vi "一体站流程质控自动启动.vi"(6 "CODMn量程切换":enum32{"H", "L", "AUTO"}(ring)=enum."AUTO", 8 "总磷量程切换":enum32{"H", "L", "AUTO"}(ring)=enum."AUTO", 9 "总氮量程切换":enum32{"H", "L", "AUTO"}(ring)=enum."AUTO", 10 "氨氮量程切换":enum32{"H", "L", "AUTO"}(ring)=enum."AUTO", 11 "参数":T1={"是否启用仪器"=FALSE, "CODMn"={"启动测量模式"={"测量模式"=enum."水样测量"}, "确定按钮"=TRUE}, "启动模块"={"氨氮"=FALSE, "总磷"=FALSE, "总氮"=FALSE, "COD"=FALSE}, "常规启动"=FALSE, "直接启动"=FALSE}) -> ()   [LabVIEW 2016, in "质控单元.lvlib"]
uses:
  PLC/PLC.lvlib
panel:
  out "枚举 2":enum16{"初始化", "采配水启动", "等待", "配水", "排水", "结束"}(ring)
  out "枚举":enum16{"初始化", "采配水启动", "等待", "配水", "排水", "结束"}(ring)
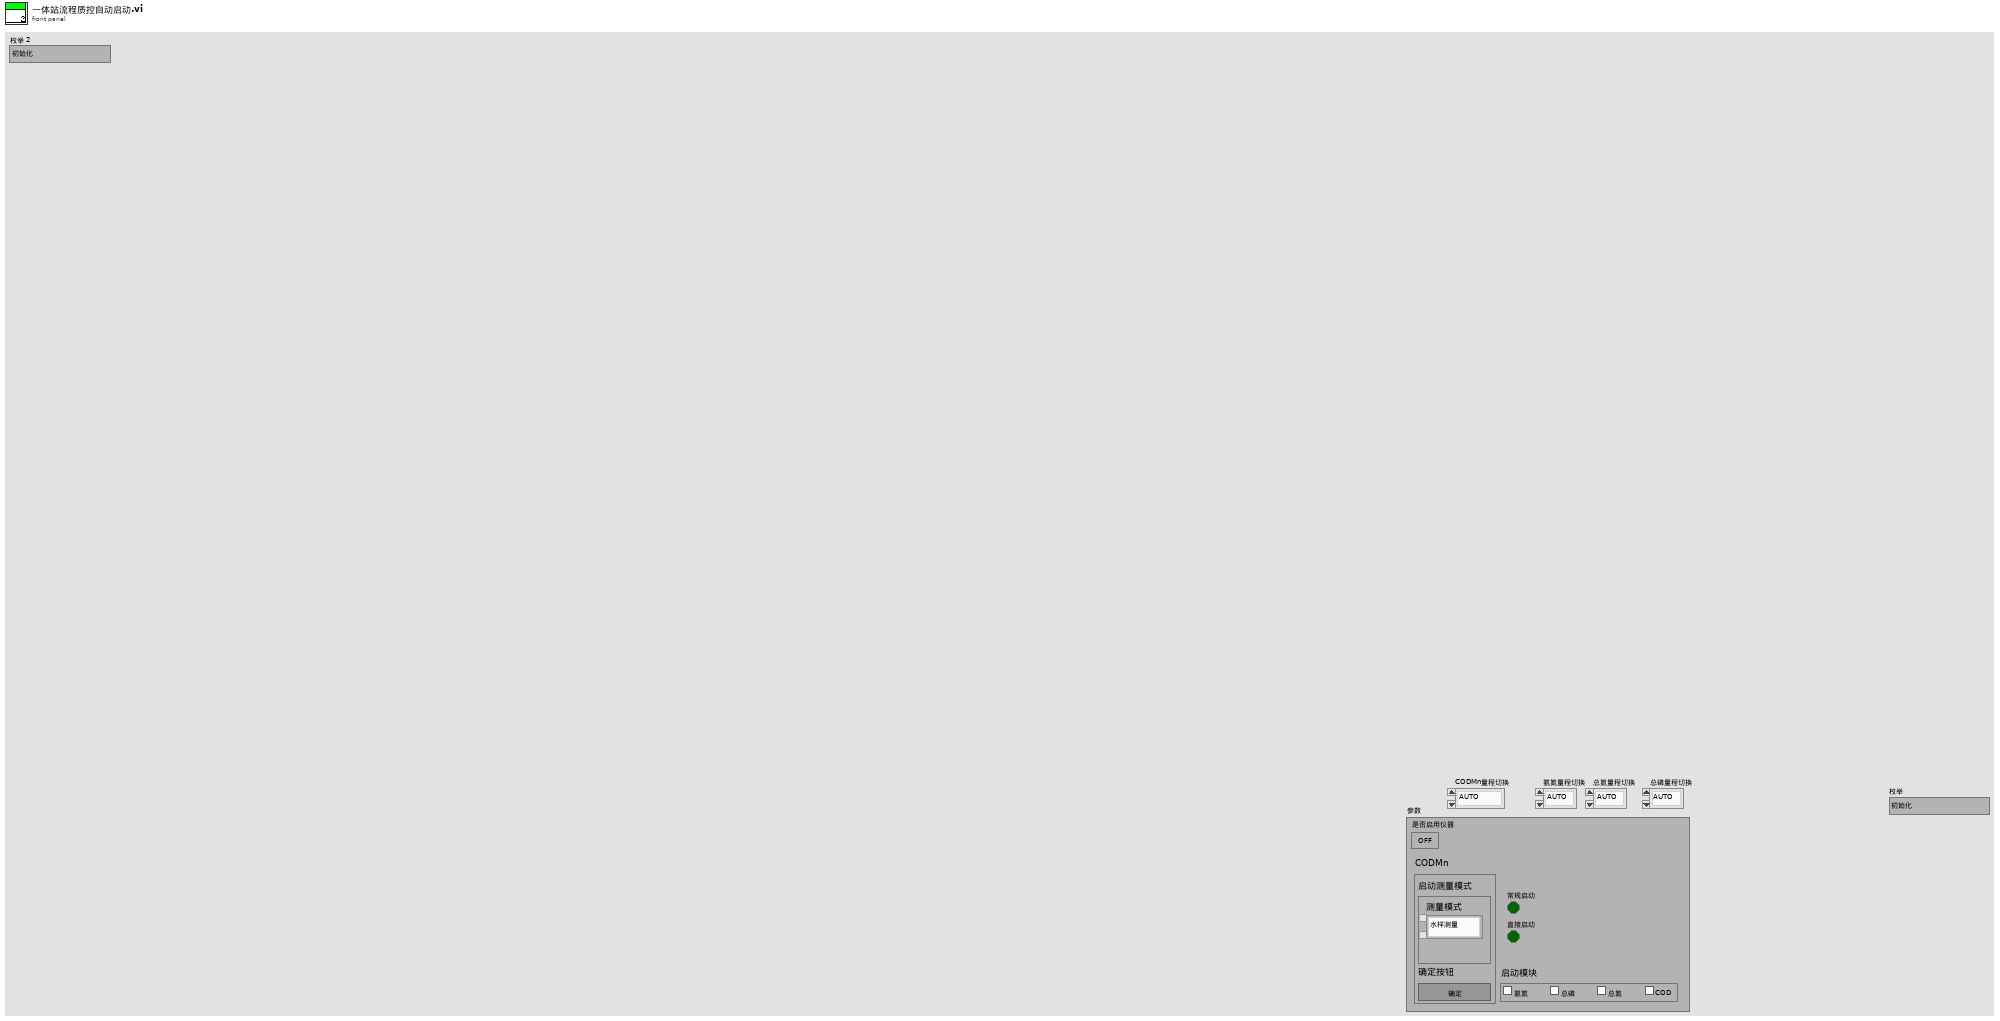
[diagram p1: front panel]
types:
  T1 = cluster{"是否启用仪器":bool, "CODMn":cluster{"启动测量模式":cluster{"测量模式":enum16{"水样测量", "标样核查", "加标回收", "平行样", "校零", "校标"}}, "确定按钮":bool}, "启动模块":cluster{"氨氮":bool, "总磷":bool, "总氮":bool, "COD":bool}, "常规启动":bool, "直接启动":bool}
  T2 = cluster{"命令":string, cluster{"starting address":u16, "holding register value":u16}}
  T3 = cluster{"R0":i16, "R1":i16, "R2":i16, "R3":i16, "R4":i16, "R5":i16, "R6":i16, "R7":i16, "R8":i16, "R9":i16, "R10":i16, "R11":i16, "R12":i16, "R13":i16, "R14":i16, "R15":i16, "R16":i16, "R17":i16, "R18":i16, "R19":i16, "R20":i16, "R21":i16, "R22":i16, "R23":i16, "R24":i16, "R25":i16, "R26":i16, "R27":i16, "R28":i16, "R29":i16, "R30":i16, "R31":i16, "R32":i16, "R33":i16, "R34":i16}
  T4 = enum32{"Bad", "Idle", "Run top level", "Running"}
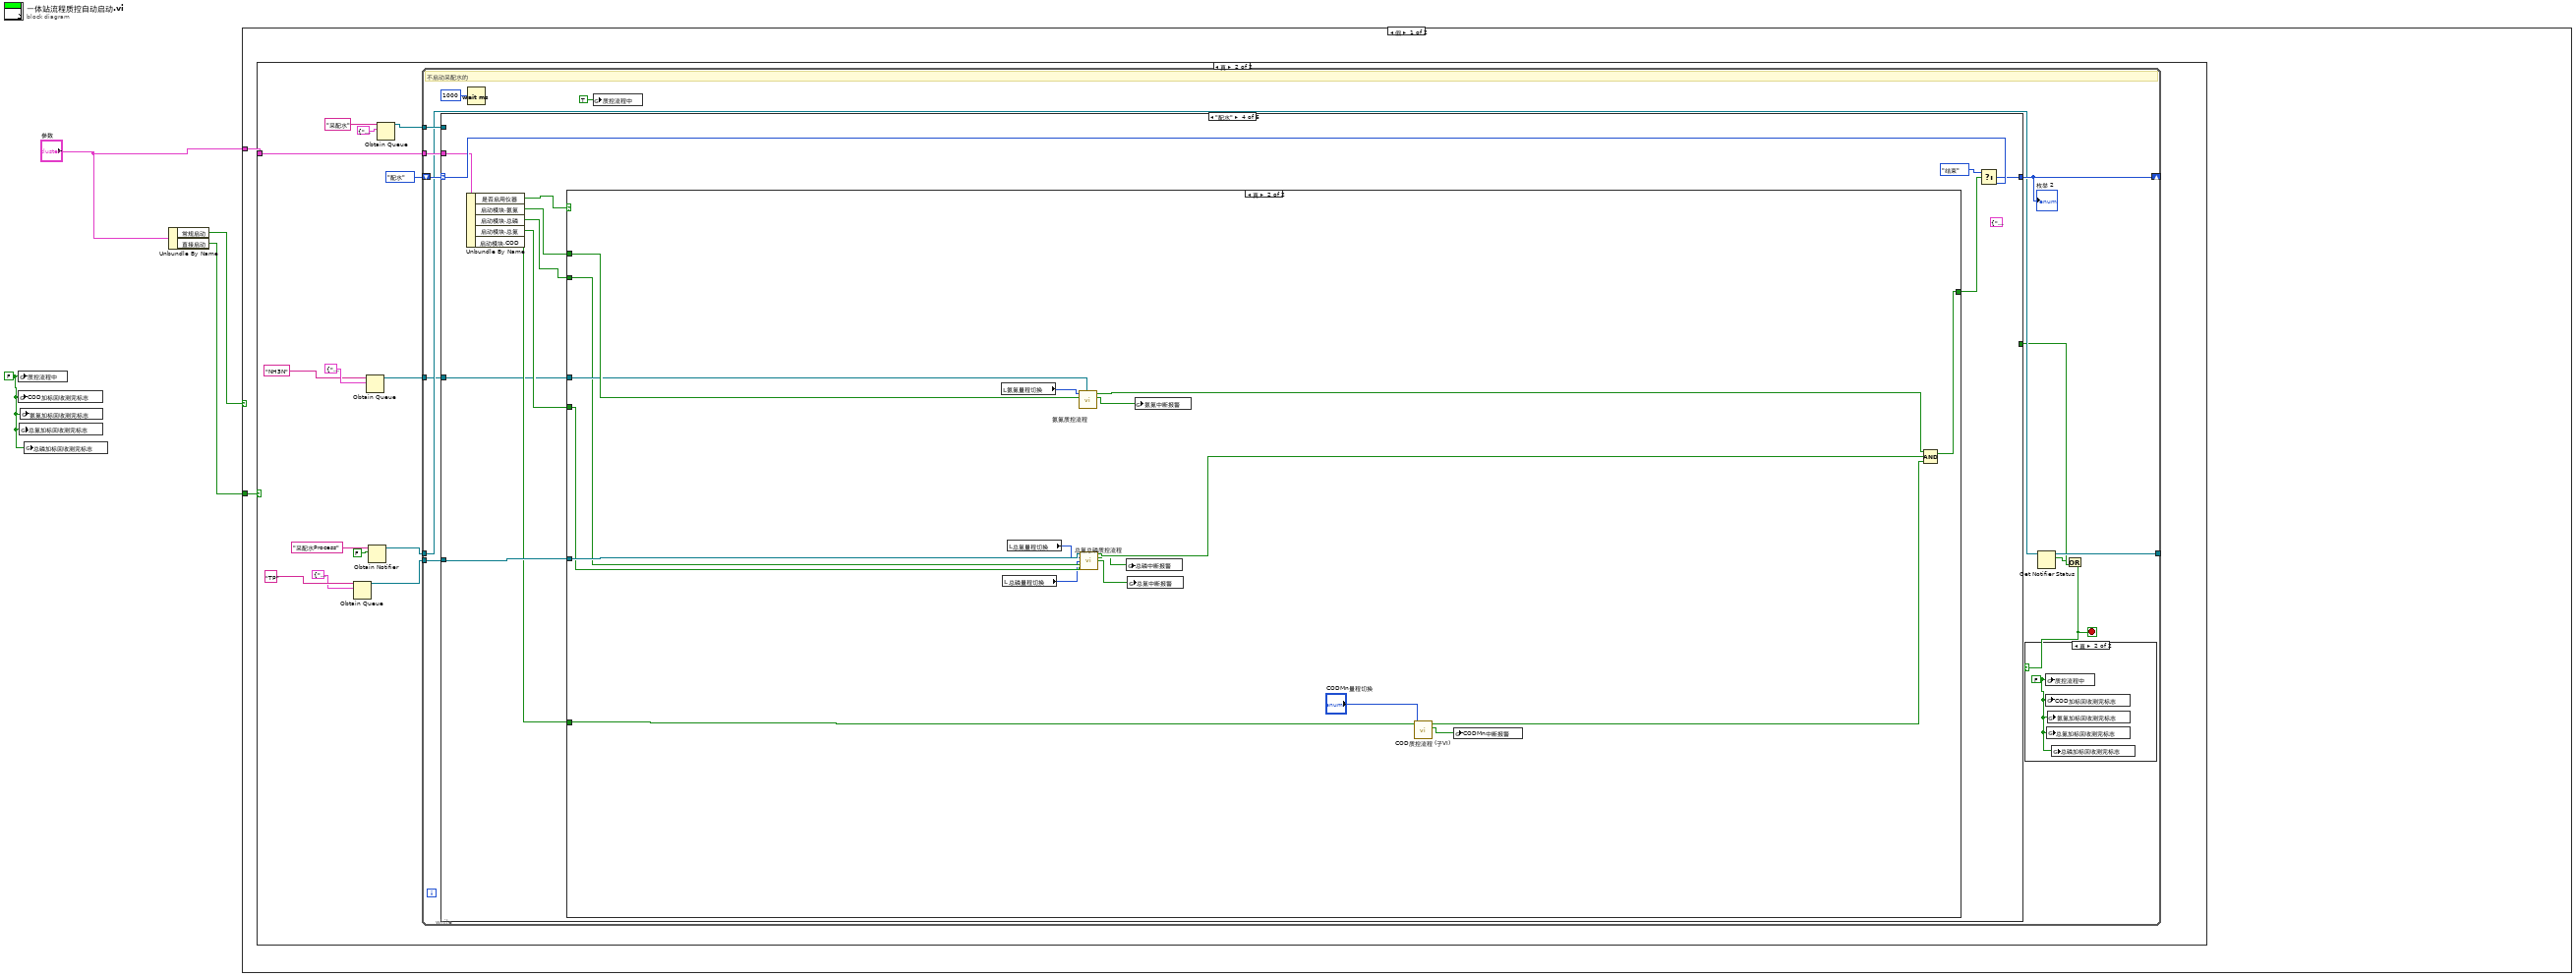
[diagram p0: block diagram]
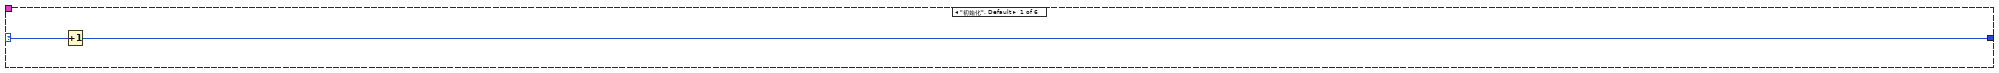
[diagram p4: hidden frame]
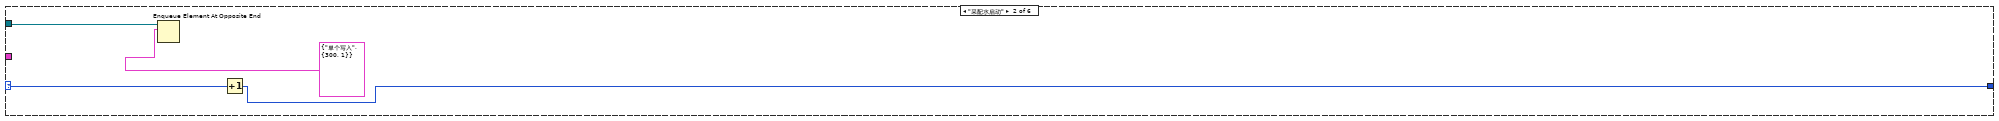
[diagram p5: hidden frame]
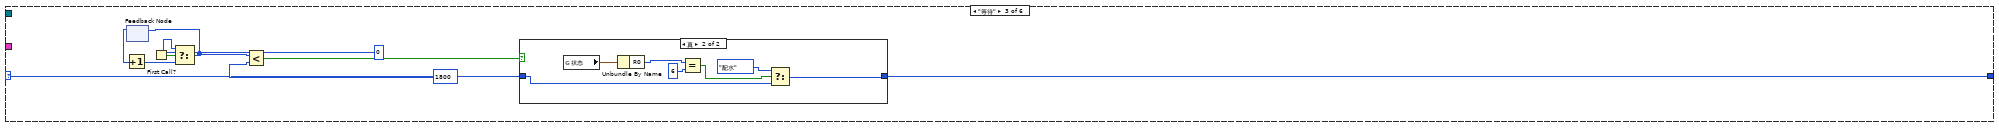
[diagram p6: hidden frame]
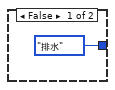
[diagram p7: hidden frame]
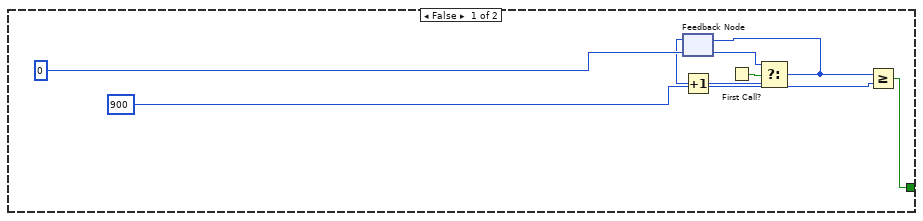
[diagram p8: hidden frame]
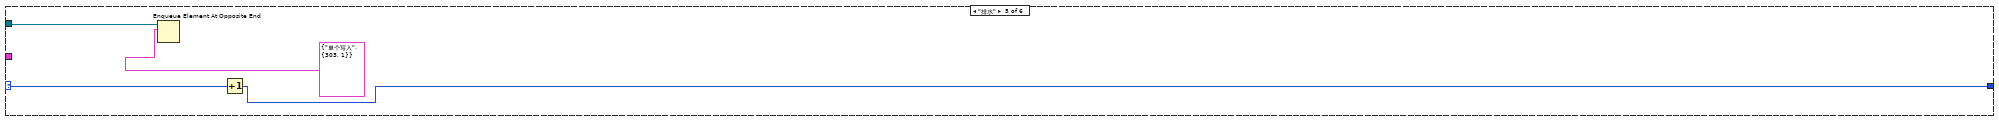
[diagram p9: hidden frame]
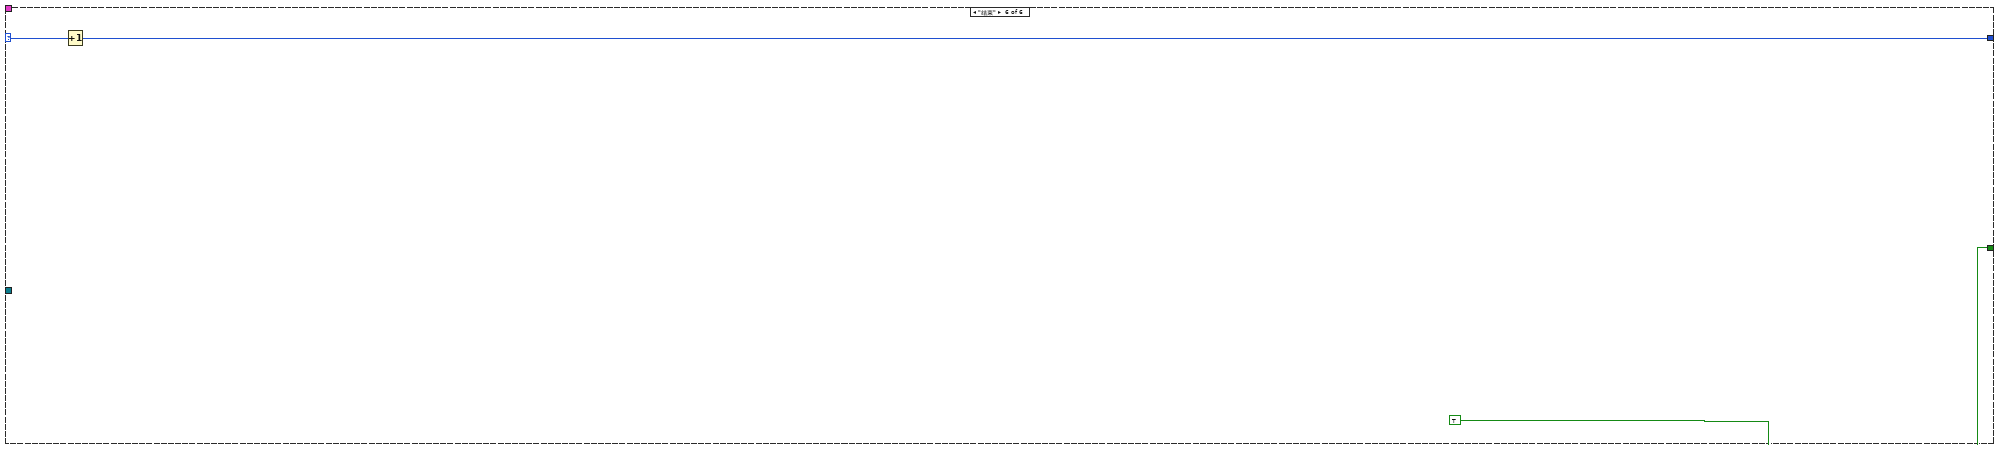
[diagram p10: hidden frame]
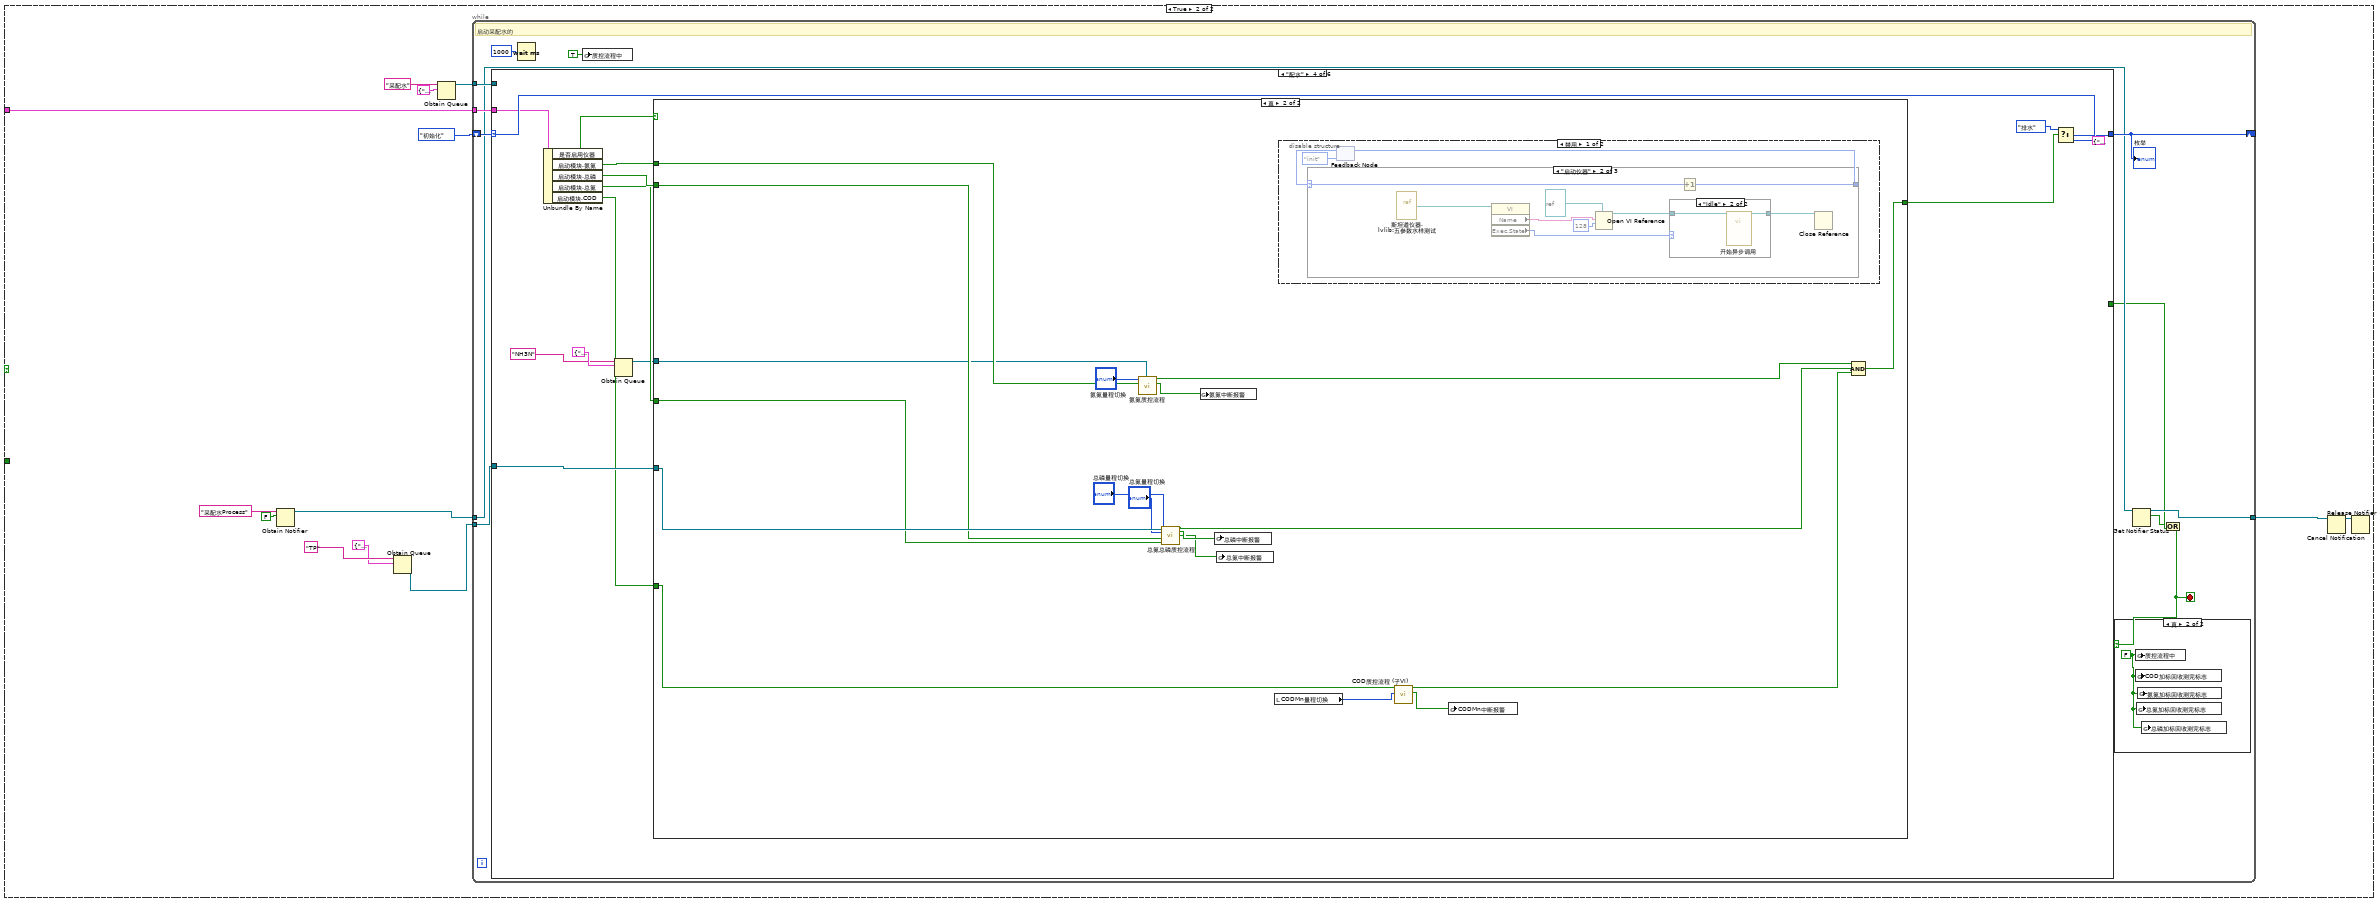
[diagram p11: hidden frame]
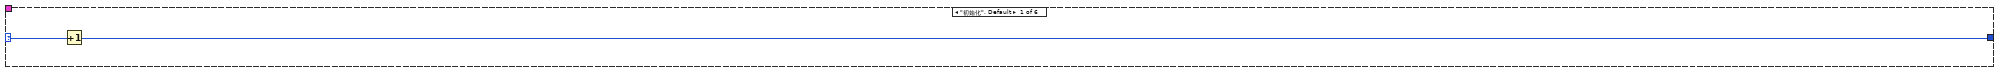
[diagram p13: hidden frame]
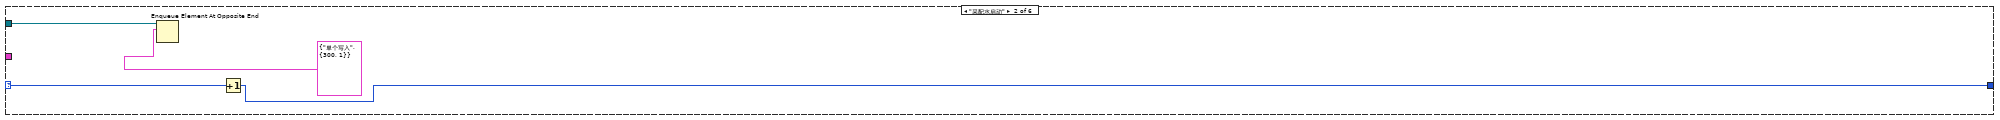
[diagram p14: hidden frame]
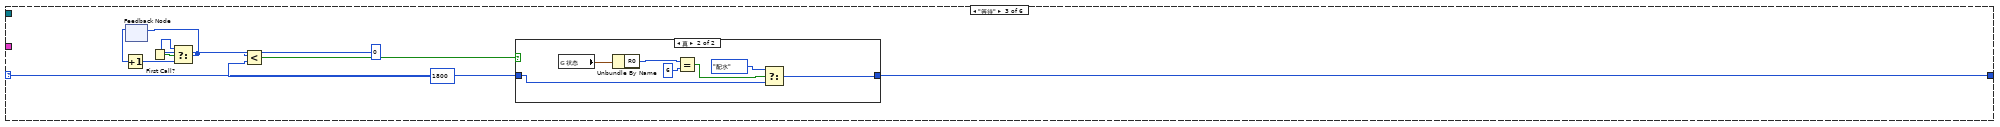
[diagram p15: hidden frame]
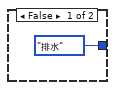
[diagram p16: hidden frame]
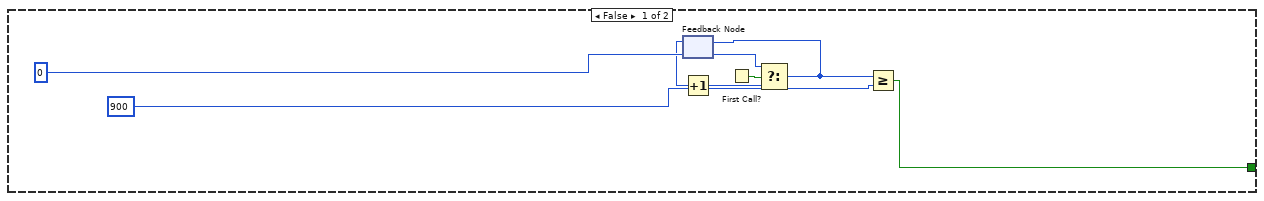
[diagram p17: hidden frame]
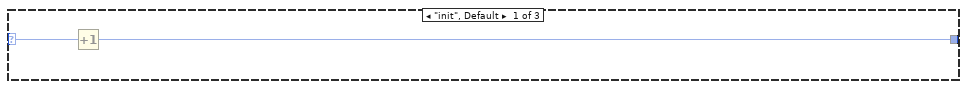
[diagram p18: hidden frame]
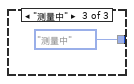
[diagram p20: hidden frame]
diagram:
  w1 = FALSE ("质控流程中")
  n1 = global write "质控测完标志全局 1.vi" "质控流程中"(w1) -> ()
  n2 = global write "质控测完标志全局 1.vi" "COD加标回收测完标志"(w1) -> ()
  n3 = global write "质控测完标志全局 1.vi" "总氮加标回收测完标志"(w1) -> ()
  n4 = global write "质控测完标志全局 1.vi" "氨氮加标回收测完标志"(w1) -> ()
  n5 = global write "质控测完标志全局 1.vi" "总磷加标回收测完标志"(w1) -> ()
  n6 = Unbundle By Name("参数") -> ("常规启动"=w3:bool, "直接启动"=w2:bool)
  n7 = case shown="假" w3 {
    tunnel: "参数" -> [w5 w102]
    tunnel: w2 -> [w6 _]
    frame False {
      n8 = case shown="真" w6 {
        tunnel: w5 -> [_ w19]
        frame False {
        }
        frame True {
          n9 = Obtain Queue(name (unnamed)="TP" ("名称（未命名）"), element data type=cluster{"命令":string, "data":variant} {"命令"="", "data"=variant}) -> (queue out=w10:refnum<queue>)  [unwired: 3 in, 2 out]
          n10 = Obtain Queue(name (unnamed)="NH3N" ("名称（未命名）"), element data type=cluster{"命令":string, "data":variant} {"命令"="", "data"=variant}) -> (queue out=w7:refnum<queue>)  [unwired: 3 in, 2 out]
          n11 = Obtain Notifier(name (unnamed)="采配水Process" ("名称（未命名）"), notification data type=FALSE) -> (notifier out=w13:refnum<notifier>)  [unwired: 2 in, 2 out]
          n12 = Obtain Queue(name (unnamed)="采配水" ("名称（未命名）"), element data type=cluster{"命令":string, "数据":variant} {"命令"="", "数据"=variant}) -> (queue out=w16:refnum<queue>)  [unwired: 3 in, 2 out]
          n13 = while {
            tunnel: w16 -> [w33]
            shift-right: [w31] -> _
            shift-left: enum16{"初始化", "采配水启动", "等待", "配水", "排水", "结束"}."配水" ("枚举") -> [w32]
            tunnel: w10 -> [w29]
            tunnel: w19 -> [w28]
            tunnel: w13 -> [w27]
            tunnel: [w26] -> _
            tunnel: w7 -> [w23]
            stop <- w22 stop-if-true
            # "不启动采配水的"
            n14 = case shown="\"配水\"" w32 {
              selector: w32 -> [w36 w38 w47 w68 w96 w101]
              tunnel: w33 -> [_ w39 _ _ w97 _]
              tunnel: [w35 w37 w46 w67 w95 w100] -> w31
              tunnel: [_ _ _ _ _ TRUE] -> w25
              tunnel: w29 -> [_ _ _ w66 _ _]
              tunnel: w28 -> [_ _ _ w63 _ _]
              tunnel: w23 -> [_ _ _ w58 _ _]
              frame "初始化", Default {
                n15 = Increment(x=w36) -> (x+1=w35:enum16{"初始化", "采配水启动", "等待", "配水", "排水", "结束"})
              }
              frame "采配水启动" {
                n16 = Enqueue Element At Opposite End(queue=w39, element=T2 {"命令"="单个写入", {"starting address"=300, "holding register value"=1}} ("元素")) -> ()  [unwired: 2 in, 3 out]
                n17 = Increment(x=w38) -> (x+1=w37:enum16{"初始化", "采配水启动", "等待", "配水", "排水", "结束"})
              }
              frame "等待" {
                n18 = feedback #1() -> (w43:i32)  [unwired: 1 in]
                n19 = Increment(x=w43) -> (x+1=w42:i32)
                n20 = First Call?() -> (First Call?: T/F=w44:bool)
                n21 = Select(t=0, s=w44, f=w42) -> (s? t:f=w41:i32)
                n22 = feedback-in #1(w41) -> ()
                n23 = Less?(x=w41, y=1800) -> (x < y?=w48:bool)
                n24 = case shown="真" w48 {
                  tunnel: w47 -> [_ w52]
                  tunnel: [enum16{"初始化", "采配水启动", "等待", "配水", "排水", "结束"}."排水" ("枚举") w51] -> w46
                  frame False {
                  }
                  frame True {
                    n25 = global read "采配水全局变量.vi" "状态"() -> (w57:T3)
                    n26 = Unbundle By Name(w57) -> ("R0"=w56:i16)
                    n27 = Equal?(x=w56, y=i16 6) -> (x = y?=w54:bool)
                    n28 = Select(t=enum16{"初始化", "采配水启动", "等待", "配水", "排水", "结束"}."配水" ("枚举"), s=w54, f=w52) -> (s? t:f=w51:enum16{"初始化", "采配水启动", "等待", "配水", "排水", "结束"})
                  }
                }
              }
              frame "配水" {
                (unwired) cluster{"命令":string, "data":variant} {"命令"="启动", "data"=variant(cluster{"站号":u16, "控制命令输出":u16[]} {"站号"=1, "控制命令输出"=[256, 0]})} ("元素")
                n29 = Unbundle By Name(w63) -> ("是否启用仪器"=w65:bool, "启动模块.氨氮"=w61:bool, "启动模块.总磷"=w62:bool, "启动模块.总氮"=w59:bool, "启动模块.COD"=w60:bool)
                n30 = case shown="真" w65 {
                  tunnel: w66 -> [_ w88]
                  tunnel: [w70 w94] -> w64
                  tunnel: w62 -> [_ w87]
                  tunnel: w61 -> [_ w93]
                  tunnel: w60 -> [_ w92]
                  tunnel: w59 -> [_ w86]
                  tunnel: w58 -> [_ w90]
                  frame False {
                    n31 = feedback #2() -> (w74:i32)  [unwired: 1 in]
                    n32 = Increment(x=w74) -> (x+1=w73:i32)
                    n33 = First Call?() -> (First Call?: T/F=w75:bool)
                    n34 = Select(t=0, s=w75, f=w73) -> (s? t:f=w71:i32)
                    n35 = feedback-in #2(w71) -> ()
                    n36 = Greater Or Equal?(x=w71, y=900) -> (x >= y?=w70:bool)
                  }
                  frame True {
                    n37 = local read "氨氮量程切换"() -> (w80:enum32{"H", "L", "AUTO"})
                    n38 = local read "总磷量程切换"() -> (w82:enum32{"H", "L", "AUTO"})
                    n39 = local read "总氮量程切换"() -> (w81:enum32{"H", "L", "AUTO"})
                    n40 = call "氨氮质控流程.vi"("队列输入NH3"=w90, "氨氮"=w93, "氨氮量程切换"=w80) -> ("氨氮中断报警"=w79:bool, "布尔"=w91:bool)  [unwired: 7 in]
                    n41 = call "总氮总磷质控流程.vi"("队列输入TP"=w88, "总氮量程切换"=w81, "总磷量程切换"=w82, "总磷"=w87, "总氮"=w86) -> ("布尔"=w85:bool, "总磷中断报警"=w78:bool, "总氮中断报警"=w77:bool)  [unwired: 8 in]
                    n42 = global write "质控中断报警全局.vi" "总磷中断报警"(w78) -> ()
                    n43 = global write "质控中断报警全局.vi" "总氮中断报警"(w77) -> ()
                    n44 = global write "质控中断报警全局.vi" "氨氮中断报警"(w79) -> ()
                    n45 = call "COD质控流程 (子VI).vi"("CODMn量程切换"="CODMn量程切换", "COD"=w92) -> ("CODMn中断报警"=w83:bool, "布尔"=w89:bool)  [unwired: 8 in]
                    n46 = global write "质控中断报警全局.vi" "CODMn中断报警"(w83) -> ()
                    n47 = Compound Arithmetic op=AND ("复合运算")(w91, w85, w89) -> (w94:bool)
                  }
                }
                n48 = Select(t=enum16{"初始化", "采配水启动", "等待", "配水", "排水", "结束"}."结束" ("枚举"), s=w64, f=w68) -> (s? t:f=w67:enum16{"初始化", "采配水启动", "等待", "配水", "排水", "结束"})
              }
              frame "排水" {
                n49 = Enqueue Element At Opposite End(queue=w97, element=T2 {"命令"="单个写入", {"starting address"=303, "holding register value"=1}} ("元素")) -> ()  [unwired: 2 in, 3 out]
                n50 = Increment(x=w96) -> (x+1=w95:enum16{"初始化", "采配水启动", "等待", "配水", "排水", "结束"})
              }
              frame "结束" {
                n51 = Increment(x=w101) -> (x+1=w100:enum16{"初始化", "采配水启动", "等待", "配水", "排水", "结束"})
              }
            }
            "枚举 2" <- w31
            n52 = Wait (ms)(milliseconds to wait=u32 1000 ("等待时间（毫秒）")) -> ()  [unwired: 1 out]
            n53 = global write "质控测完标志全局 1.vi" "质控流程中"(TRUE ("质控流程中")) -> ()
            n54 = Get Notifier Status(notifier=w27) -> (notifier out=w26:refnum<notifier>, current notification=w24:bool)  [unwired: 1 in, 3 out]
            n55 = Or(x=w24, y=w25) -> (x .or. y?=w22:bool)
            n56 = case shown="真" w22 {
              frame False {
              }
              frame True {
                w34 = FALSE ("质控流程中")
                n57 = global write "质控测完标志全局 1.vi" "质控流程中"(w34) -> ()
                n58 = global write "质控测完标志全局 1.vi" "COD加标回收测完标志"(w34) -> ()
                n59 = global write "质控测完标志全局 1.vi" "总氮加标回收测完标志"(w34) -> ()
                n60 = global write "质控测完标志全局 1.vi" "氨氮加标回收测完标志"(w34) -> ()
                n61 = global write "质控测完标志全局 1.vi" "总磷加标回收测完标志"(w34) -> ()
              }
            }
          }
        }
      }
    }
    frame True {
      n62 = Obtain Notifier(name (unnamed)="采配水Process" ("名称（未命名）"), notification data type=FALSE) -> (notifier out=w105:refnum<notifier>)  [unwired: 2 in, 2 out]
      n63 = Obtain Queue(name (unnamed)="TP" ("名称（未命名）"), element data type=cluster{"命令":string, "data":variant} {"命令"="", "data"=variant}) -> (queue out=w108:refnum<queue>)  [unwired: 3 in, 2 out]
      n64 = Obtain Queue(name (unnamed)="采配水" ("名称（未命名）"), element data type=cluster{"命令":string, "数据":variant} {"命令"="", "数据"=variant}) -> (queue out=w112:refnum<queue>)  [unwired: 3 in, 2 out]
      n65 = while {
        tunnel: w112 -> [w126]
        shift-right: [w124] -> _
        shift-left: enum16{"初始化", "采配水启动", "等待", "配水", "排水", "结束"}."初始化" ("枚举") -> [w125]
        tunnel: w108 -> [w122]
        tunnel: w102 -> [w121]
        tunnel: w105 -> [w120]
        tunnel: [w119] -> w104
        stop <- w116 stop-if-true
        # "启动采配水的"
        n66 = case shown="\"配水\"" w125 {
          selector: w125 -> [w129 w131 w140 w163 w209 w214]
          tunnel: w126 -> [_ w132 _ _ w210 _]
          tunnel: [w128 w130 w139 w162 w208 w213] -> w124
          tunnel: [_ _ _ _ _ TRUE] -> w118
          tunnel: w122 -> [_ _ _ w161 _ _]
          tunnel: w121 -> [_ _ _ w158 _ _]
          frame "初始化", Default {
            n67 = Increment(x=w129) -> (x+1=w128:enum16{"初始化", "采配水启动", "等待", "配水", "排水", "结束"})
          }
          frame "采配水启动" {
            n68 = Enqueue Element At Opposite End(queue=w132, element=T2 {"命令"="单个写入", {"starting address"=300, "holding register value"=1}} ("元素")) -> ()  [unwired: 2 in, 3 out]
            n69 = Increment(x=w131) -> (x+1=w130:enum16{"初始化", "采配水启动", "等待", "配水", "排水", "结束"})
          }
          frame "等待" {
            n70 = feedback #3() -> (w136:i32)  [unwired: 1 in]
            n71 = Increment(x=w136) -> (x+1=w135:i32)
            n72 = First Call?() -> (First Call?: T/F=w137:bool)
            n73 = Select(t=0, s=w137, f=w135) -> (s? t:f=w134:i32)
            n74 = feedback-in #3(w134) -> ()
            n75 = Less?(x=w134, y=1800) -> (x < y?=w141:bool)
            n76 = case shown="真" w141 {
              tunnel: w140 -> [_ w145]
              tunnel: [enum16{"初始化", "采配水启动", "等待", "配水", "排水", "结束"}."排水" ("枚举") w144] -> w139
              frame False {
              }
              frame True {
                n77 = global read "采配水全局变量.vi" "状态"() -> (w150:T3)
                n78 = Unbundle By Name(w150) -> ("R0"=w149:i16)
                n79 = Equal?(x=w149, y=i16 6) -> (x = y?=w147:bool)
                n80 = Select(t=enum16{"初始化", "采配水启动", "等待", "配水", "排水", "结束"}."配水" ("枚举"), s=w147, f=w145) -> (s? t:f=w144:enum16{"初始化", "采配水启动", "等待", "配水", "排水", "结束"})
              }
            }
          }
          frame "配水" {
            (unwired) cluster{"命令":string, "data":variant} {"命令"="启动", "data"=variant(cluster{"站号":u16, "控制命令输出":u16[]} {"站号"=1, "控制命令输出"=[256, 0]})} ("元素")
            n81 = Unbundle By Name(w158) -> ("是否启用仪器"=w160:bool, "启动模块.氨氮"=w156:bool, "启动模块.总磷"=w157:bool, "启动模块.总氮"=w154:bool, "启动模块.COD"=w155:bool)
            n82 = Obtain Queue(name (unnamed)="NH3N" ("名称（未命名）"), element data type=cluster{"命令":string, "data":variant} {"命令"="", "data"=variant}) -> (queue out=w151:refnum<queue>)  [unwired: 3 in, 2 out]
            n83 = case shown="真" w160 {
              tunnel: w161 -> [_ w184]
              tunnel: [w165 w188] -> w159
              tunnel: w157 -> [_ w183]
              tunnel: w156 -> [_ w187]
              tunnel: w155 -> [_ w186]
              tunnel: w154 -> [_ w182]
              tunnel: w151 -> [_ w180]
              frame False {
                n84 = feedback #4() -> (w169:i32)  [unwired: 1 in]
                n85 = Increment(x=w169) -> (x+1=w168:i32)
                n86 = First Call?() -> (First Call?: T/F=w170:bool)
                n87 = Select(t=0, s=w170, f=w168) -> (s? t:f=w166:i32)
                n88 = feedback-in #4(w166) -> ()
                n89 = Greater Or Equal?(x=w166, y=900) -> (x >= y?=w165:bool)
              }
              frame True {
                n90 = call "氨氮质控流程.vi"("队列输入NH3"=w180, "氨氮"=w187, "氨氮量程切换"="氨氮量程切换") -> ("氨氮中断报警"=w172:bool, "布尔"=w189:bool)  [unwired: 7 in]
                n91 = call "总氮总磷质控流程.vi"("队列输入TP"=w184, "总氮量程切换"="总氮量程切换", "总磷量程切换"="总磷量程切换", "总磷"=w183, "总氮"=w182) -> ("布尔"=w181:bool, "总磷中断报警"=w174:bool, "总氮中断报警"=w173:bool)  [unwired: 8 in]
                n92 = global write "质控中断报警全局.vi" "氨氮中断报警"(w172) -> ()
                n93 = global write "质控中断报警全局.vi" "总磷中断报警"(w174) -> ()
                n94 = global write "质控中断报警全局.vi" "总氮中断报警"(w173) -> ()
                n95 = local read "CODMn量程切换"() -> (w179:enum32{"H", "L", "AUTO"})
                n96 = disable-structure shown="禁用" {
                  frame Disabled {
                    n97 = feedback #5(enum16{"init", "启动仪器", "测量中"}."init") -> (w191:enum16{"init", "启动仪器", "测量中"})
                    n98 = case shown="\"启动仪器\"" w191 {
                      selector: w191 -> [w194 w203 _]
                      tunnel: [w193 w202 enum16{"init", "启动仪器", "测量中"}."测量中"] -> w192
                      frame "init", Default {
                        n99 = Increment(x=w194) -> (x+1=w193:enum16{"init", "启动仪器", "测量中"})
                      }
                      frame "启动仪器" {
                        n100 = vi-ref "斯坦道仪器.lvlib:五参数水样测试.vi"() -> (w195:refnum<vi>)
                        n101 = property class="VI"(reference=w195) -> ("Name"=w199:string, "Exec.State"=w197:T4)  [unwired: 1 in, 2 out]
                        n102 = Open VI Reference(type specifier VI Refnum (for type only)=refnum<vi> refnum ("类型说明符VI引用句柄（仅用于类型）"), vi path=w199, options=128 ("选项")) -> (vi reference=w198:refnum<vi>)  [unwired: 3 in, 1 out]
                        n103 = case shown="\"Idle\"" w197 {
                          tunnel: w198 -> [w204 w206]
                          tunnel: [w204 w205] -> w196
                          frame "Bad", Default {
                          }
                          frame "Idle" {
                            n104 = call-by-ref "开始异步调用"(reference=w206) -> (reference out=w205:refnum<vi>)  [unwired: 13 in, 1 out]
                          }
                        }
                        n105 = Increment(x=w203) -> (x+1=w202:enum16{"init", "启动仪器", "测量中"})
                        n106 = Close Reference(reference=w196) -> ()  [unwired: 1 in, 1 out]
                      }
                      frame "测量中" {
                      }
                    }
                    n107 = feedback-in #5(w192) -> ()
                  }
                  frame Enabled {
                  }
                }
                n108 = call "COD质控流程 (子VI).vi"("CODMn量程切换"=w179, "COD"=w186) -> ("CODMn中断报警"=w178:bool, "布尔"=w185:bool)  [unwired: 8 in]
                n109 = global write "质控中断报警全局.vi" "CODMn中断报警"(w178) -> ()
                n110 = Compound Arithmetic op=AND ("复合运算")(w189, w181, w185) -> (w188:bool)
              }
            }
            n111 = Select(t=enum16{"初始化", "采配水启动", "等待", "配水", "排水", "结束"}."排水" ("枚举"), s=w159, f=w163) -> (s? t:f=w162:enum16{"初始化", "采配水启动", "等待", "配水", "排水", "结束"})
          }
          frame "排水" {
            n112 = Enqueue Element At Opposite End(queue=w210, element=T2 {"命令"="单个写入", {"starting address"=303, "holding register value"=1}} ("元素")) -> ()  [unwired: 2 in, 3 out]
            n113 = Increment(x=w209) -> (x+1=w208:enum16{"初始化", "采配水启动", "等待", "配水", "排水", "结束"})
          }
          frame "结束" {
            n114 = Increment(x=w214) -> (x+1=w213:enum16{"初始化", "采配水启动", "等待", "配水", "排水", "结束"})
          }
        }
        "枚举" <- w124
        n115 = Wait (ms)(milliseconds to wait=u32 1000 ("等待时间（毫秒）")) -> ()  [unwired: 1 out]
        n116 = global write "质控测完标志全局 1.vi" "质控流程中"(TRUE ("质控流程中")) -> ()
        n117 = Get Notifier Status(notifier=w120) -> (notifier out=w119:refnum<notifier>, current notification=w117:bool)  [unwired: 1 in, 3 out]
        n118 = Or(x=w117, y=w118) -> (x .or. y?=w116:bool)
        n119 = case shown="真" w116 {
          frame False {
          }
          frame True {
            w127 = FALSE ("质控流程中")
            n120 = global write "质控测完标志全局 1.vi" "质控流程中"(w127) -> ()
            n121 = global write "质控测完标志全局 1.vi" "COD加标回收测完标志"(w127) -> ()
            n122 = global write "质控测完标志全局 1.vi" "总氮加标回收测完标志"(w127) -> ()
            n123 = global write "质控测完标志全局 1.vi" "氨氮加标回收测完标志"(w127) -> ()
            n124 = global write "质控测完标志全局 1.vi" "总磷加标回收测完标志"(w127) -> ()
          }
        }
      }
      n125 = Cancel Notification(0:w104) -> (8:w103:refnum<notifier>)  [unwired: 1 in, 2 out]
      n126 = Release Notifier(notifier=w103) -> ()  [unwired: 2 in, 3 out]
    }
  }
